vi "CredentialLogin.vi"(8 "error in (no error)":errorcluster) -> (0 "error out":errorcluster, 1 "LoggedIn?":bool, 2 "Timeout?":bool, 3 "UserName":string)   [LabVIEW 2019]
uses:
  <vilib>/event_ctls.llb/eventvkey.ctl
panel:
  in  "Password":string
  in  "User Name":string
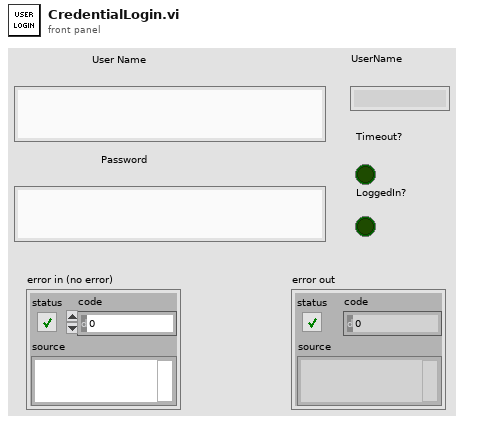
[diagram p1: front panel]
types:
  T1 = typedef "eventvkey.ctl" = enum16{"ASCII", "Enter", "Return", "Shift", "Ctrl", "Alt", "Cmd", "Opt", "Caps", "NumLock", "Clear", "Break", "Up", "Down", "Left", "Right", "Insert", "Delete", "Home", "End", "PageUp", "PageDown", "Escape", "Help", "Pause", "ScrollLock", "F1", "F2", "F3", "F4", "F5", "F6", "F7", "F8", "F9", "F10", "F11", "F12", "F13", "F14", "F15", "F16", "F17", "F18", "F19", "F20", "F21", "F22", "F23", "F24", "Play", "VolumeUp", "VolumeDown", "Mute", "Two Byte Char"}
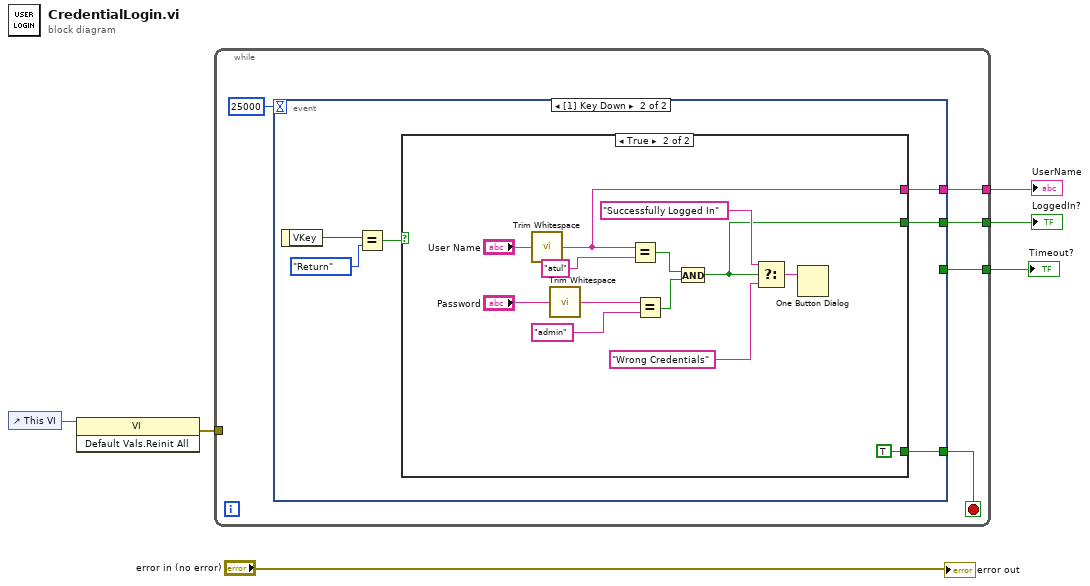
[diagram p0: block diagram]
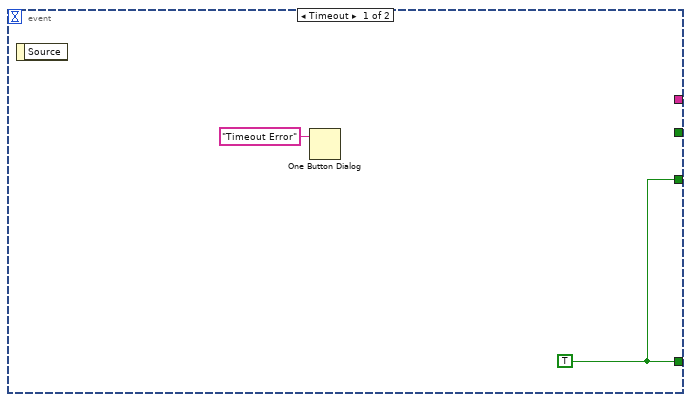
[diagram p2: hidden frame]
diagram:
  n1 = control-ref of="This VI"() -> (w2:refnum<vi>)
  n2 = invoke class="VI" method="Default Vals.Reinit All"(reference=w2) -> (error out=w1:errorcluster)  [unwired: 2 in, 2 out]
  n3 = while {
    tunnel: [w9] -> w6
    tunnel: [w8] -> w5
    tunnel: [w7] -> w4
    tunnel: w1 -> [_]
    stop <- w10 stop-if-true
    n4 = event shown="[1] Key Down" {
      selector: _ -> [_ _]
      dyn-events: _ -> [_ _]
      timeout: 25000 -> [_ _]
      tunnel: [w13 w15] -> w10
      tunnel: [w13 _] -> w9
      tunnel: [_ w16] -> w8
      tunnel: [_ w14] -> w7
      event Timeout {
        w13 = TRUE
        n5 = event-data() -> ()  [unwired: 1 in, 1 out]
        n6 = One Button Dialog(message="Timeout Error") -> ()  [unwired: 1 in, 1 out]
      }
      event Key Down {
        n7 = event-data() -> ("VKey"=w19:T1)  [unwired: 1 in]
        n8 = Equal?(x=w19, y=eventvkey."Return") -> (x = y?=w17:bool)
        n9 = case shown="True" w17 {
          tunnel: [_ w25] -> w16
          tunnel: [_ TRUE] -> w15
          tunnel: [_ w23] -> w14
          frame False {
          }
          frame True {
            n10 = call <vilib>:"Trim Whitespace.vi"("string"="User Name") -> ("trimmed string"=w23:string)  [unwired: 1 in]
            n11 = call <vilib>:"Trim Whitespace.vi"("string"="Password") -> ("trimmed string"=w20:string)  [unwired: 1 in]
            n12 = Equal?(x=w23, y="atul") -> (x = y?=w30:bool)
            n13 = Equal?(x=w20, y="admin") -> (x = y?=w29:bool)
            n14 = And(x=w30, y=w29) -> (x .and. y?=w25:bool)
            n15 = Select(t="Successfully Logged In" ("y"), s=w25, f="Wrong Credentials" ("y")) -> (s? t:f=w26:string)
            n16 = One Button Dialog(message=w26) -> ()  [unwired: 1 in, 1 out]
          }
        }
      }
    }
  }
  "Timeout?" <- w6
  "LoggedIn?" <- w5
  "UserName" <- w4
  "error out" <- "error in (no error)"
